vi "UTILITY Elapsed Time.vi"(6 "precision (6)":i16=6, 7 "Add Elapsed Time (hrs)":bool, 8 "error in (no error)":errorcluster, 11 "Reset Timer":bool) -> (0 "error out":errorcluster, 1 "Main Loop Rate":dbl format="%0.2f", 2 "Elapsed Time":dbl, 3 "Total Array":string[][](array[string]), 5 "Main Start":dbl format="%.2f")   [LabVIEW 2023]
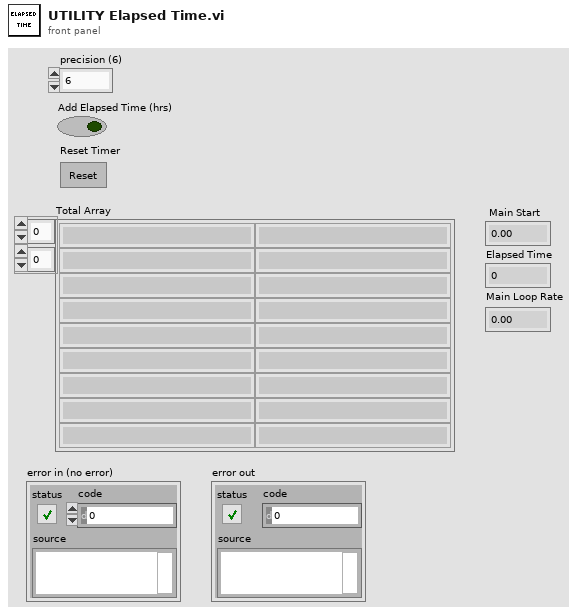
[diagram p1: front panel]
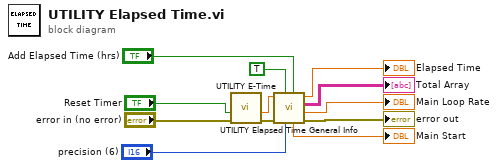
[diagram p0: block diagram]
diagram:
  n1 = call "UTILITY E-Time.vi"("error in (no error)"="error in (no error)", "Reset"="Reset Timer") -> ("error out"=w5:errorcluster, "Elapsed Time (sec)"=w12:dbl)  [unwired: 7 in, 1 out]
  n2 = call "UTILITY Elapsed Time General Info.vi"("Add Elapsed Time (hrs)"="Add Elapsed Time (hrs)", "precision (6)"="precision (6)", "Add Software Elapsed Time"=TRUE, "Error In"=w5, "Elapsed Time (sec)"=w12) -> ("Error Out"=→"error out":errorcluster, "Main Loop Rate"=→"Main Loop Rate":dbl, "Total Array"=→"Total Array":string[][], "Elapsed Time"=→"Elapsed Time":dbl, "Main Start"=→"Main Start":dbl)  [unwired: 2 in]
